vi "Test Dashboard.vi"() -> ()   [LabVIEW 2016]
uses:
  Program Files (x86)/National Instruments/LabVIEW 2016/examples/robotics/EPOS2 CANOpen Driver/Low Level VIs/Typedefs/FPGA CAN Frame Cluster.ctl
  BMS Status.ctl
  RT/Battery Status.ctl
  <vilib>/Utility/miscctls.llb/LVRowAndColumnUnsignedTypeDef.ctl
  <vilib>/Platform/TimedLoop/XDataNode/timing_clust.ctl
  <vilib>/Platform/TimedLoop/XDataNode/nitl_modes.ctl
  <vilib>/Platform/TimedLoop/XDataNode/wakeup.ctl
  RT/Read All CAN.vi
  RT/Data to BMS Status.vi
  RT/Data to Battery Status.vi
  <vilib>/Platform/TimedLoop/XDataNode/XDataNode.xnode
  <vilib>/Platform/TimedLoop/XDataNode/XDNodeRunTimeDep.lvlib
panel:
  in  "Tab Control":enum32{"Play!", "Debugg"}(tab)
  in  "Boot into load sequence":bool
  in  "No load":bool
  in  "Enter Stage":bool
  in  "Enter precharge":bool
  out "BMS Status":T1
  out "Stage req status":u8[](array[numeric])
  out "Stage req updates":u16
  out "Errors updates":u16
  out "Errors":u8[][](array[numeric]) format="%x"
  out "Battery Status":T2
  in  "CAN Frame":T3={"Timestamp"=0, "Identifier"=0, "Type"=0, "InfoA"=0, "InfoB"=0, "DataLength"=0, "Data"=[0, 0, 0, 0, 0, 0, 0, 0]} {"Data" format="%.0x"; "DataLength" format="%.0x"; "InfoB" format="%.0x"; "InfoA" format="%.0x"; "Type" format="%.0x"; "Identifier" format="%.0x"; "Timestamp" format="%.0x"}
  in  "Send once":bool
  in  "Send cont.":bool
  in  "Stop":bool
  out "Error Out":errorcluster
  out "CAN Frame Out":T3 {"Data" format="%.0x"; "DataLength" format="%.0x"; "InfoB" format="%.0x"; "InfoA" format="%.0x"; "Type" format="%.0x"; "Identifier" format="%.0x"; "Timestamp" format="%.0x"}
  in  "Clear list":bool
  out "Multicolumn Listbox":i32(listbox)
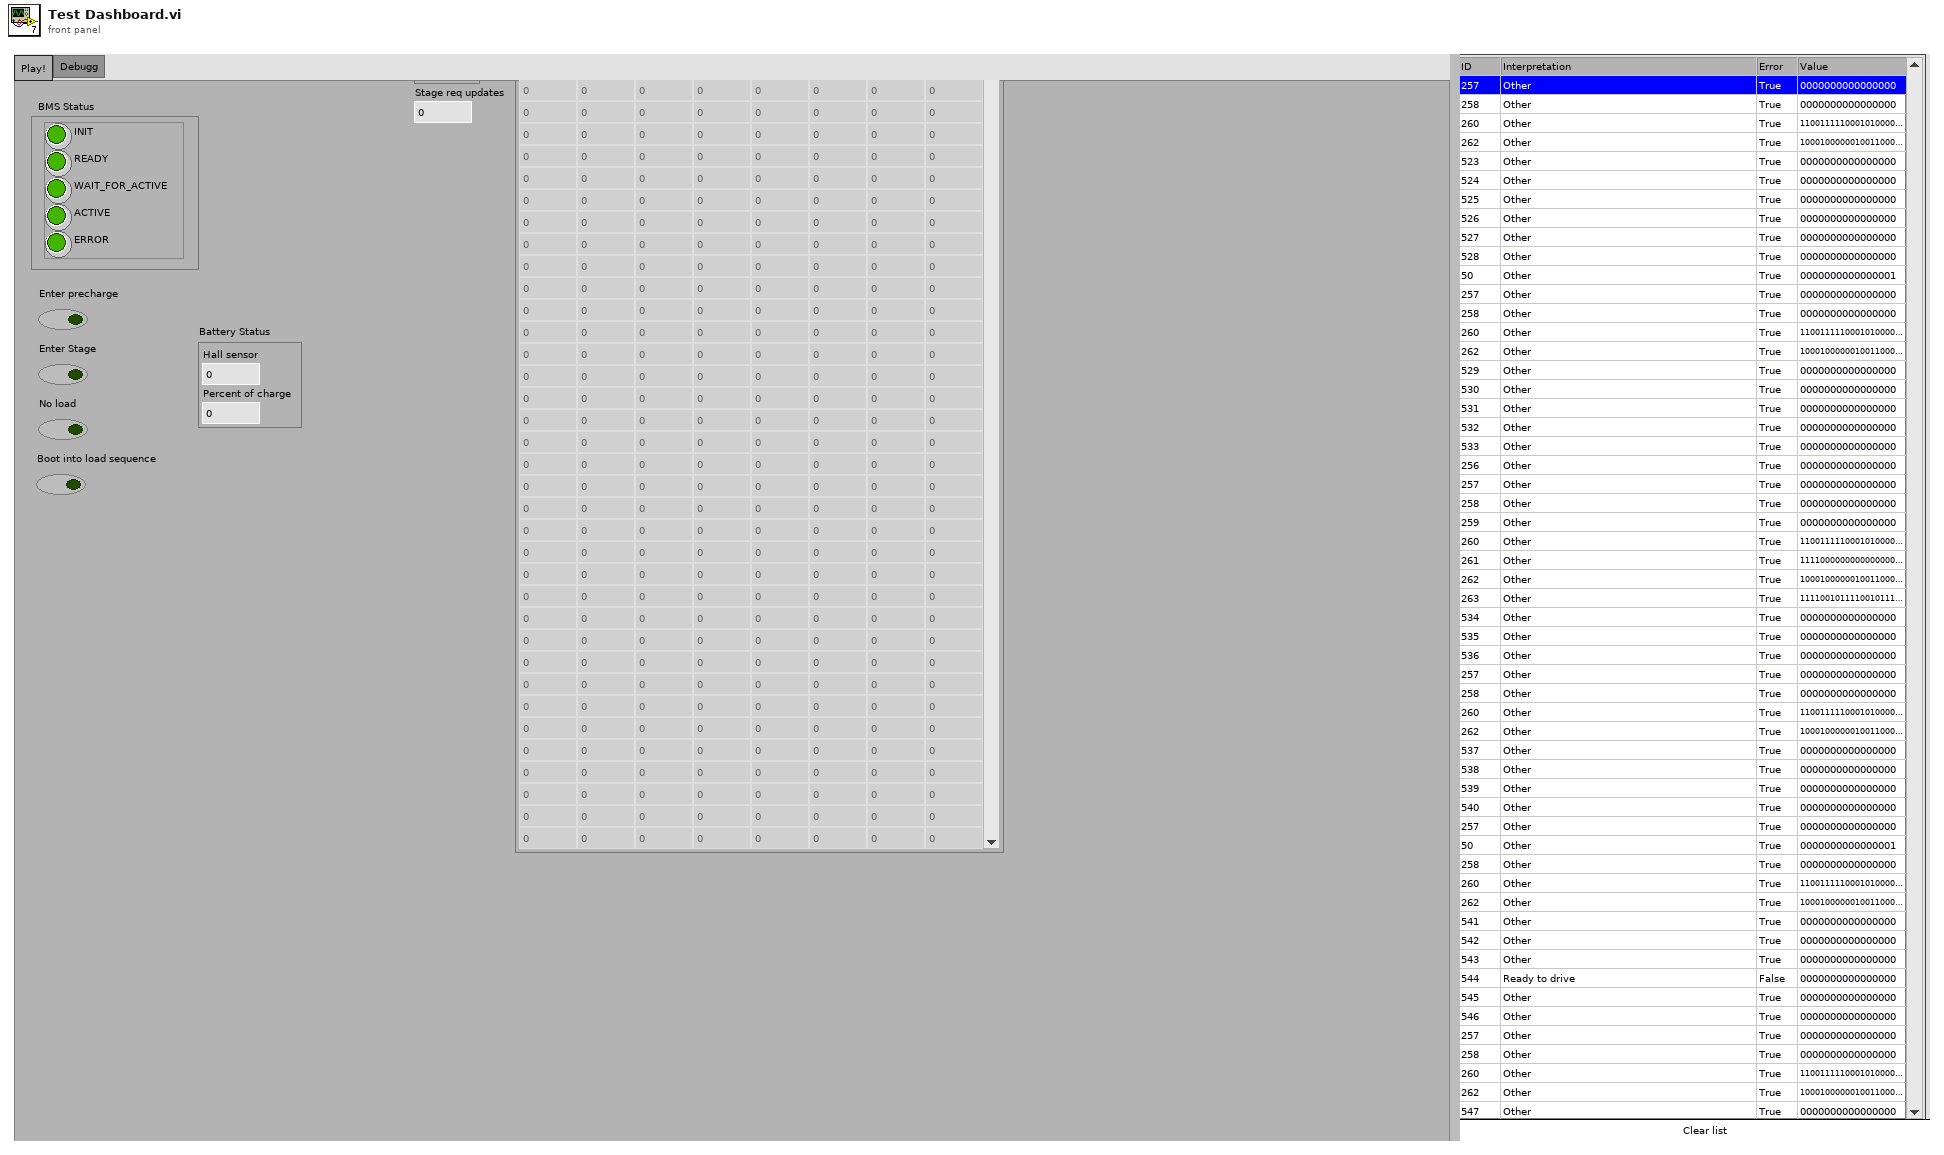
[diagram p1: front panel]
types:
  T1 = typedef "BMS Status.ctl" = cluster{"INIT":bool, "READY":bool, "WAIT_FOR_ACTIVE":bool, "ACTIVE":bool, "ERROR":bool}
  T2 = typedef "Battery Status.ctl" = cluster{"Hall sensor":i32, "Percent of charge":i16}
  T3 = typedef "FPGA CAN Frame Cluster.ctl" = cluster{"Timestamp":u64, "Identifier":u32, "Type":u8, "InfoA":u8, "InfoB":u8, "DataLength":u8, "Data":u8[]}
  T4 = cluster{"Message":string, "ID":u16, "Error":bool}[]
  T5 = typedef "XDNodeRunTimeDep.lvlib/timing_clust.ctl" = cluster{"Expected End [f-1]":u64, "Actual End [f-1]":u64, "Finished Late? [f-1]":bool, "Expected End [i-1]":u64, "Actual End [i-1]":u64, "Finished Late? [i-1]":bool, "Expected Start [i]":u64, "Actual Start [i]":u64, "Expected Start [f]":u64, "Actual Start [f]":u64, "Source Name":string, "Structure Name":string, "Period":i64, "Deadline":i64, "Offset":i64, "Start":i64, "Priority":i32, "Timeout":i32, "Mode":T6, "Wakeup Reason":T7, "Error":errorcluster, "Source Type":string, "Secondary Source Type":string, "Global End Time":u64, "Global Start Time":u64, "Frame Duration":u64, "Iteration Duration":u64, "Assigned CPU":i32, "I/O Scan Engine Mode":u32}
  T6 = typedef "XDNodeRunTimeDep.lvlib/nitl_modes.ctl" = enum32{"No Change", "Process missed periods, maintain original phase", "Discard missed periods, maintain original phase", "Process missed periods, ignore original phase", "Discard missed periods, ignore original phase"}
  T7 = typedef "XDNodeRunTimeDep.lvlib/wakeup.ctl" = enum32{"Normal", "Aborted", "Asynchronous wakeup", "Timing source error", "Timed loop error", "Timeout"}
  T8 = typedef "LVRowAndColumnUnsignedTypeDef.ctl" = cluster{"Row":u32, "Column":u32}
  T9 = typedef "CAN Refnum.ctl" = refnum<k1>
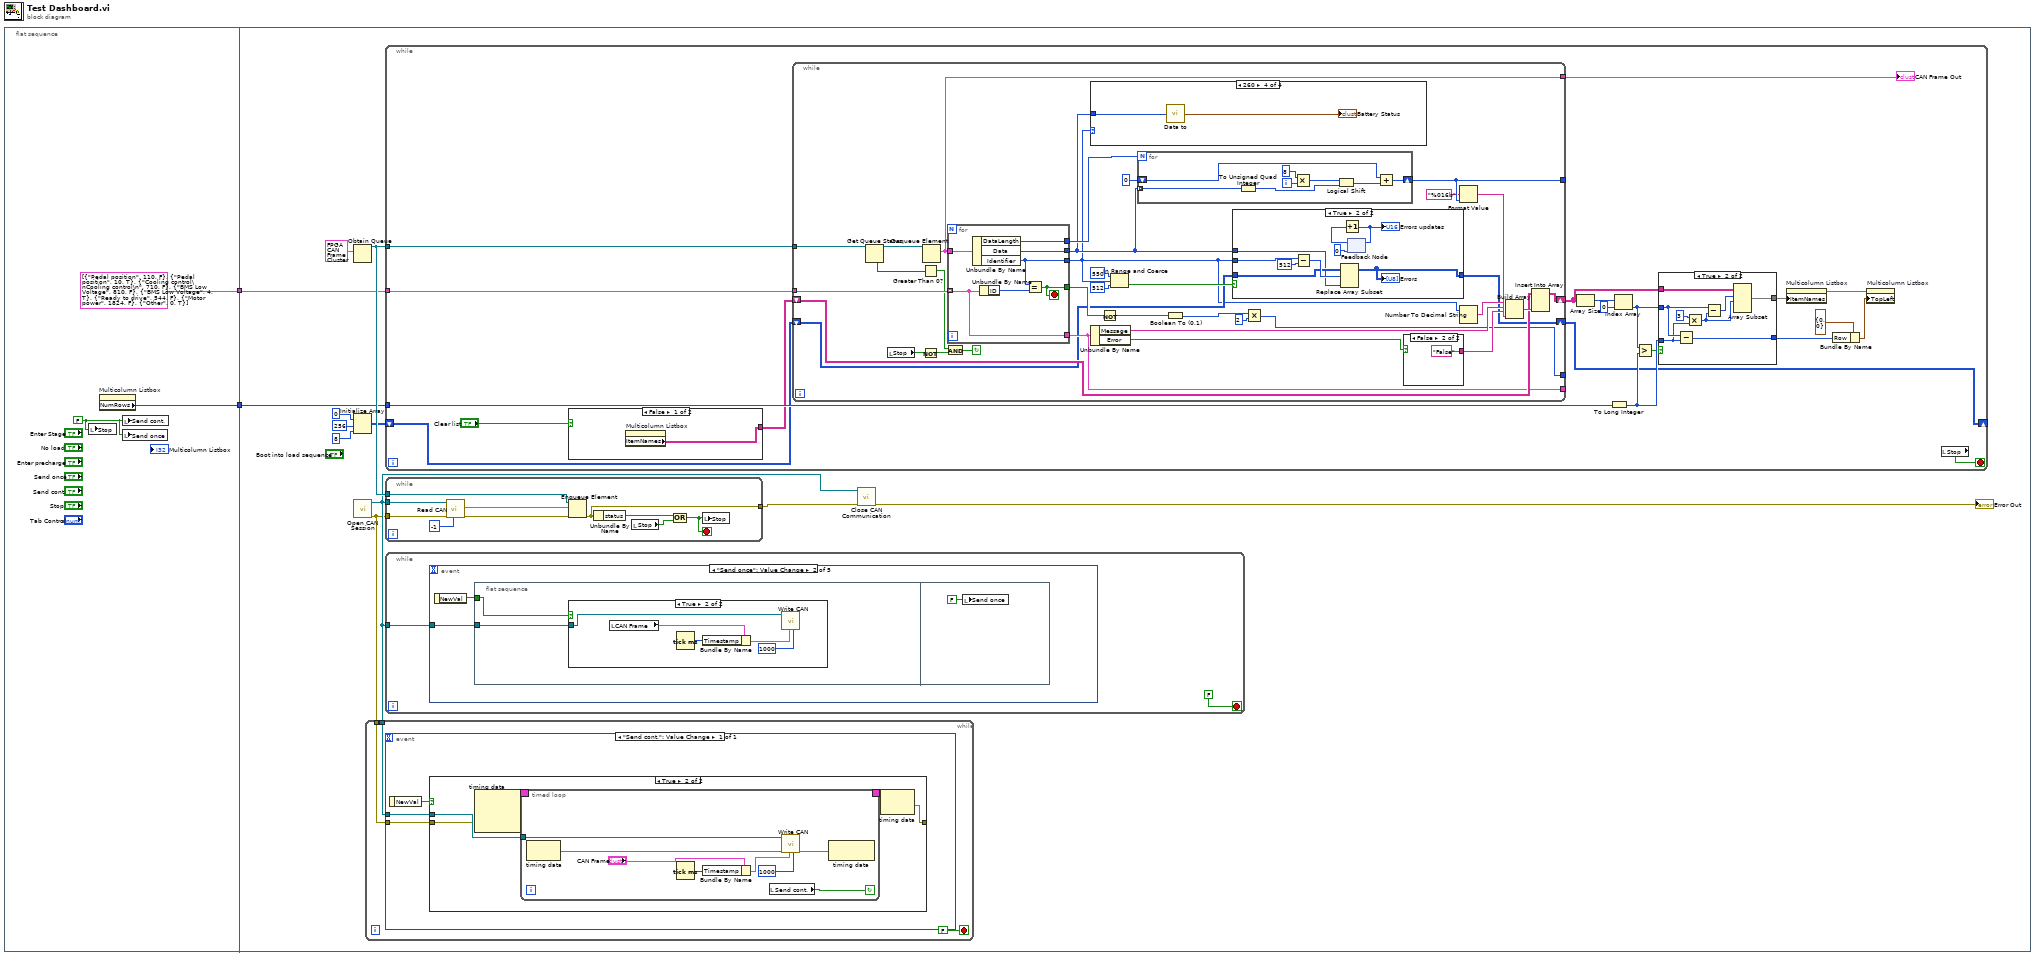
[diagram p0: block diagram]
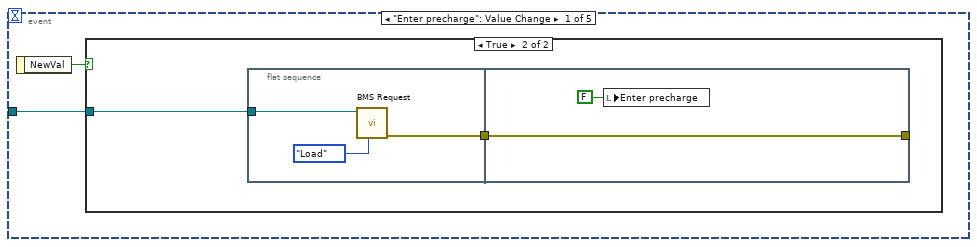
[diagram p3: hidden frame]
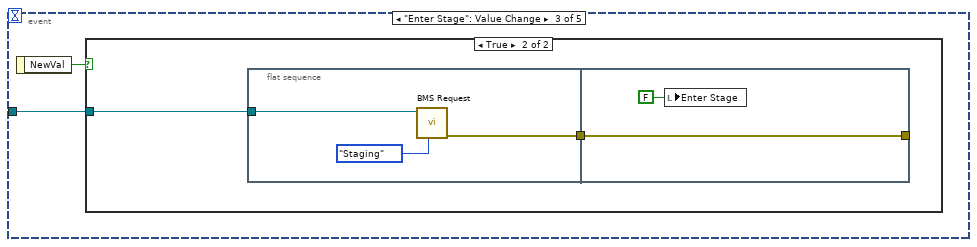
[diagram p6: hidden frame]
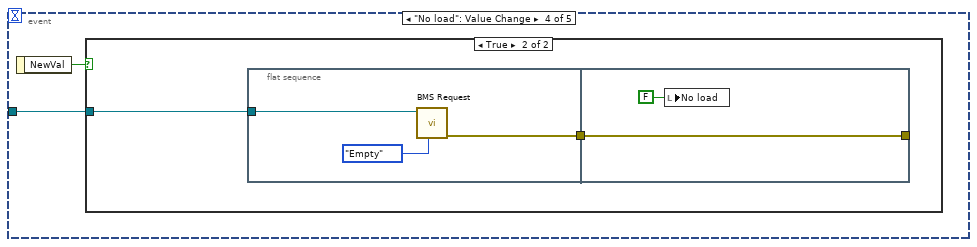
[diagram p8: hidden frame]
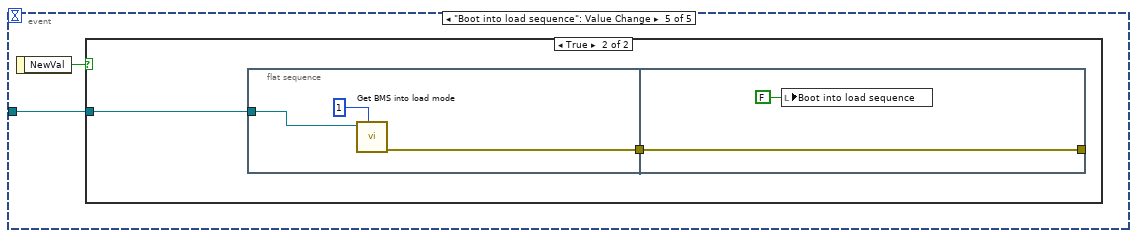
[diagram p10: hidden frame]
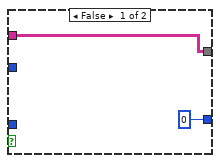
[diagram p12: hidden frame]
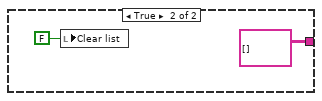
[diagram p13: hidden frame]
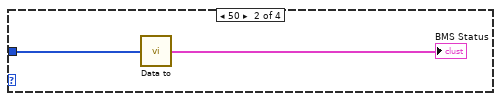
[diagram p16: hidden frame]
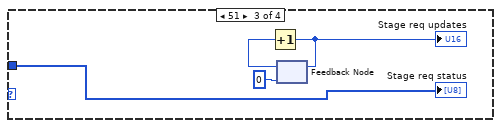
[diagram p17: hidden frame]
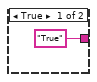
[diagram p18: hidden frame]
diagram:
  n1 = flat-sequence {
    tunnel: [w4] -> w2
    tunnel: [T4 [{"Message"="Pedal position", "ID"=110, "Error"=FALSE}, {"Message"="Pedal position", "ID"=10, "Error"=TRUE}, {"Message"="Cooling control\nCooling control\n", "ID"=710, "Error"=FALSE}, {"Message"="BMS Low Voltage", "ID"=810, "Error"=FALSE}, {"Message"="BMS Low Voltage", "ID"=4, "Error"=TRUE}, {"Message"="Ready to drive", "ID"=544, "Error"=FALSE}, {"Message"="Motor power", "ID"=1824, "Error"=FALSE}, {"Message"="Other", "ID"=0, "Error"=TRUE}] ("Messages")] -> w1
    tunnel: w2 -> [w14]
    tunnel: w1 -> [w13]
    frame #0 {
      w5 = FALSE
      n2 = local write "Stop"(w5) -> ()
      n3 = property on="Multicolumn Listbox" class="MCListbox (strict)"() -> ("NumRows"=w4:u32)  [unwired: 2 in, 2 out]
      n4 = local write "Send cont."(w5) -> ()
      n5 = local write "Send once"(w5) -> ()
    }
    frame #1 {
      n6 = Initialize Array(u8 0 ("element"), 256 ("dimension size"), 8 ("dimension size")) -> (w9:u8[][])
      n7 = Obtain Queue(element data type=T3 {"Timestamp"=0, "Identifier"=0, "Type"=0, "InfoA"=0, "InfoB"=0, "DataLength"=0, "Data"=[0, 0, 0, 0, 0, 0, 0, 0]} ("CAN Frame Out")) -> (queue out=w16:refnum<queue>)  [unwired: 4 in, 2 out]
      n8 = call "Open CAN Session.vi"() -> ("error out"=w6:errorcluster, "CAN Session"=w7:T9)  [unwired: 10 in]
      n9 = while {
        tunnel: w7 -> [w20]
        tunnel: w6 -> [w19]
        stop <- FALSE stop-if-true
        n10 = event shown="[0] \"Send cont.\": Value Change" {
          selector: _ -> [_]
          dyn-events: _ -> [_]
          timeout: _ -> [_]
          tunnel: w20 -> [w22]
          tunnel: w19 -> [w21]
          event "Send cont.": Value Change {
            n11 = event-data() -> ("NewVal"=w23:bool)  [unwired: 1 in]
            n12 = case shown="True" w23 {
              tunnel: w21 -> [w24 w26]
              tunnel: w22 -> [_ w27]
              tunnel: [w24 w25] -> _
              frame False {
              }
              frame True {
                n13 = node-c288(w26) -> (w29:T5)  [unwired: 2 in]
                n14 = timed-loop {
                  timing: w29 -> [_]
                  timing-out: [_] -> w28
                  tunnel: w27 -> [w37]
                  stop <- w34 continue-if-true
                  n15 = node-c288() -> (w36:errorcluster)  [unwired: 1 in]
                  n16 = Tick Count (ms)() -> (millisecond timer value=w30:u32)
                  n17 = Bundle By Name(cluster="CAN Frame", "Timestamp"=w30) -> (w31:T3)
                  n18 = local read "Send cont."() -> (w34:bool)
                  n19 = call "Write CAN.vi"("timeout"=1000, "CAN Frame"=w31, "error in"=w36, "CAN Session In"=w37) -> ("error out"=w35:errorcluster)  [unwired: 6 in, 1 out]
                  n20 = node-c288(w35) -> ()  [unwired: 1 out]
                }
                n21 = node-c288(w28) -> (w25:errorcluster)
              }
            }
          }
        }
      }
      n22 = while {
        tunnel: w16 -> [w115]
        tunnel: w14 -> [w109]
        tunnel: w13 -> [w108]
        shift-right: [w96] -> _
        shift-left: w9 -> [w97]
        stop <- w113 stop-if-true
        n23 = case shown="False" "Clear list" {
          tunnel: [w126 string[][] [] ("Item Names")] -> w106
          frame False {
            n24 = property on="Multicolumn Listbox" class="MCListbox (strict)"() -> ("ItemNames"=w126:string[][])  [unwired: 2 in, 2 out]
          }
          frame True {
            n25 = local write "Clear list"(FALSE) -> ()
          }
        }
        n26 = while {
          tunnel: w115 -> [w160]
          tunnel: [w145] -> _
          tunnel: [w137] -> _
          tunnel: [w144] -> w114
          tunnel: [w143] -> _
          shift-right: [w146] -> w102
          shift-left: w106 -> [w147]
          tunnel: w108 -> [w142]
          shift-right: [w131] -> w96
          shift-left: w97 -> [w132]
          stop <- w138 continue-if-true
          n27 = Get Queue Status(queue=w160) -> (queue out=w161:refnum<queue>, # elements in queue=w162:i32)  [unwired: 2 in, 6 out]
          n28 = local read "Stop"() -> (w141:bool)
          n29 = Greater Than 0?(x=w162) -> (x > 0?=w139:bool)
          n30 = Not(x=w141) -> (.not. x?=w140:bool)
          n31 = Dequeue Element(queue=w161) -> (element=w144:T3)  [unwired: 2 in, 3 out]
          n32 = And(x=w139, y=w140) -> (x .and. y?=w138:bool)
          n33 = for {
            tunnel: w142 -> [w195] mode=indexing
            tunnel: w144 -> [w197]
            tunnel: [w195] -> w143
            tunnel: [w194] -> w149
            tunnel: [w193] -> w130
            tunnel: [w192] -> w148
            tunnel: [w191] -> w129
            stop <- w194 stop-if-true
            n34 = Unbundle By Name(w197) -> ("DataLength"=w192:u8, "Data"=w193:u8[], "Identifier"=w191:u32)
            n35 = Unbundle By Name(w195) -> ("ID"=w196:u16)
            n36 = Equal?(x=w191, y=w196) -> (x = y?=w194:bool)
          }
          n37 = case shown="260" w129 {
            tunnel: w130 -> [_ w174 w178 w180]
            frame 0, Default {
            }
            frame 50 {
              n38 = call-poly "Data to.vi"("Data"=w174) -> ("BMS Status"=→"BMS Status":T1)
            }
            frame 51 {
              n39 = feedback #1(u16 0) -> (w177:u16)
              n40 = Increment(x=w177) -> (x+1=w176:u16)
              "Stage req updates" <- w176
              n41 = feedback-in #1(w176) -> ()
              "Stage req status" <- w178
            }
            frame 260 {
              n42 = call-poly "Data to.vi"("Data"=w180) -> ("Battery Status"=→"Battery Status":T2)
            }
          }
          n43 = Unbundle By Name(w143) -> ("Message"=w153:string, "Error"=w155:bool)
          n44 = Not(x=w149) -> (.not. x?=w152:bool)
          n45 = In Range and Coerce(upper limit=u16 550, x=w129, lower limit=u16 512) -> (In Range?=w133:bool)  [unwired: 1 out]
          n46 = for {
            N: w148 -> [_]
            shift-right: [w182] -> w137
            shift-left: u64 0 -> [w184]
            tunnel: w130 -> [w181] mode=indexing
            i -> [w186]
            n47 = To Unsigned Quad Integer(1:w181) -> (0:w183:u64)
            n48 = Multiply(x=i8 8, y=w186) -> (x*y=w185:i32)
            n49 = Logical Shift(y=w185, x=w183) -> (x << y=w188:u64)
            n50 = Add(x=w184, y=w188) -> (x+y=w182:u64)
          }
          n51 = Boolean To (0,1)(Boolean=w152) -> (0, 1=w150:i16)
          n52 = case shown="True" w133 {
            tunnel: w132 -> [w163 w167]
            tunnel: [w163 w166] -> w131
            tunnel: w130 -> [_ w165]
            tunnel: w129 -> [_ w164]
            frame False {
            }
            frame True {
              n53 = Subtract(x=w164, y=u32 512) -> (x-y=w172:u32)
              n54 = Replace Array Subset(array=w167, new element=w165, index (row)=w172) -> (w166:u8[][])  [unwired: 1 in]
              "Errors" <- w166
              n55 = feedback #2(u16 0) -> (w168:u16)
              n56 = Increment(x=w168) -> (x+1=w169:u16)
              "Errors updates" <- w169
              n57 = feedback-in #2(w169) -> ()
            }
          }
          n58 = Multiply(x=w150, y=i16 2) -> (x*y=w145:i16)
          n59 = case shown="False" w155 {
            tunnel: ["True" "False"] -> w156
            frame True {
            }
            frame False {
            }
          }
          n60 = Format Value(format string="%016b", value (0)=w137) -> (output string=w158:string)  [unwired: 1 in]
          n61 = Number To Decimal String(number=w129) -> (decimal integer string=w154:string)  [unwired: 1 in]
          n62 = Build Array(w154, w153, w156, w158) -> (w157:string[])
          n63 = Insert Into Array(array=w147, new element=w157) -> (w146:string[][])  [unwired: 2 in]
        }
        "CAN Frame Out" <- w114
        n64 = Array Size(array=w102) -> (size(s)=w104:i32[])
        n65 = To Long Integer(number=w109) -> (32bit integer=w99:i32)
        n66 = Index Array(array=w104, index=0) -> (element=w100:i32)
        n67 = Greater?(x=w100, y=w99) -> (0:w98:bool)
        n68 = case shown="True" w98 {
          tunnel: [0 w118] -> w103
          tunnel: w99 -> [_ w119]
          tunnel: w100 -> [_ w120]
          tunnel: w102 -> [w116 w123]
          tunnel: [w116 w122] -> w101
          frame False {
          }
          frame True {
            n69 = Subtract(x=w120, y=w119) -> (x-y=w118:i32)
            n70 = Multiply(x=3, y=w119) -> (x*y=w124:i32)
            n71 = Subtract(x=w120, y=w124) -> (x-y=w125:i32)
            n72 = Array Subset(array=w123, index (row)=w125, length (row)=w124) -> (w122:string[][])  [unwired: 2 in]
          }
        }
        n73 = property on="Multicolumn Listbox" class="MCListbox (strict)"("ItemNames"=w101) -> (error out=w105:errorcluster)  [unwired: 2 in, 1 out]
        n74 = Bundle By Name(cluster=T8 {"Row"=0, "Column"=0} ("Top Left Visible Cell"), "Row"=w103) -> (w112:T8)
        n75 = property on="Multicolumn Listbox" class="MCListbox (strict)"(error in=w105, "TopLeft"=w112) -> ()  [unwired: 1 in, 2 out]
        n76 = local read "Stop"() -> (w113:bool)
      }
      n77 = while {
        tunnel: w6 -> [w199]
        tunnel: w7 -> [w198]
        tunnel: w16 -> [w205]
        tunnel: [w203] -> w15
        stop <- w206 stop-if-true
        n78 = call-poly "Read CAN.vi"("timeout in ms (-1)"=-1, "error in"=w199, "CAN Session In"=w198) -> ("error out"=w201:errorcluster, "CAN Frame Out"=w202:T3)  [unwired: 6 in, 1 out]
        n79 = Enqueue Element(queue=w205, element=w202, error in (no error)=w201) -> (error out=w203:errorcluster)  [unwired: 1 in, 2 out]
        n80 = Unbundle By Name(w203) -> ("status"=w204:bool)
        n81 = local read "Stop"() -> (w207:bool)
        n82 = Or(x=w204, y=w207) -> (x .or. y?=w206:bool)
        n83 = local write "Stop"(w206) -> ()
      }
      n84 = while {
        tunnel: w7 -> [w49]
        stop <- FALSE stop-if-true
        n85 = event shown="[1] \"Send once\": Value Change" {
          selector: _ -> [_ _ _ _ _]
          dyn-events: _ -> [_ _ _ _ _]
          timeout: _ -> [_ _ _ _ _]
          tunnel: w49 -> [w51 w59 w70 w79 w88]
          event "Enter precharge": Value Change {
            n86 = event-data() -> ("NewVal"=w50:bool)  [unwired: 1 in]
            n87 = case shown="True" w50 {
              tunnel: w51 -> [_ w52]
              frame False {
              }
              frame True {
                n88 = flat-sequence {
                  tunnel: [w55] -> w53
                  tunnel: w52 -> [w56]
                  tunnel: [w58] -> _
                  tunnel: w53 -> [w58]
                  frame #0 {
                    n89 = call "BMS Request.vi"("Request"=enum16{"Empty", "Load", "Staging"}."Load", "CAN Session In"=w56) -> ("error out"=w55:errorcluster)  [unwired: 8 in, 1 out]
                  }
                  frame #1 {
                    n90 = local write "Enter precharge"(FALSE) -> ()
                  }
                }
              }
            }
          }
          event "Send once": Value Change {
            n91 = event-data() -> ("NewVal"=w60:bool)  [unwired: 1 in]
            n92 = flat-sequence {
              tunnel: w60 -> [w62]
              tunnel: w59 -> [w61]
              frame #0 {
                n93 = case shown="True" w62 {
                  tunnel: w61 -> [_ w63]
                  frame False {
                  }
                  frame True {
                    n94 = local read "CAN Frame"() -> (w64:T3)
                    n95 = Tick Count (ms)() -> (millisecond timer value=w65:u32)
                    n96 = Bundle By Name(cluster=w64, "Timestamp"=w65) -> (w66:T3)
                    n97 = call "Write CAN.vi"("timeout"=1000, "CAN Frame"=w66, "CAN Session In"=w63) -> ()  [unwired: 7 in, 2 out]
                  }
                }
              }
              frame #1 {
                n98 = local write "Send once"(FALSE ("Send once")) -> ()
              }
            }
          }
          event "Enter Stage": Value Change {
            n99 = event-data() -> ("NewVal"=w69:bool)  [unwired: 1 in]
            n100 = case shown="True" w69 {
              tunnel: w70 -> [_ w71]
              frame False {
              }
              frame True {
                n101 = flat-sequence {
                  tunnel: [w74] -> w72
                  tunnel: w71 -> [w75]
                  tunnel: [w77] -> _
                  tunnel: w72 -> [w77]
                  frame #0 {
                    n102 = call "BMS Request.vi"("Request"=enum16{"Empty", "Load", "Staging"}."Staging", "CAN Session In"=w75) -> ("error out"=w74:errorcluster)  [unwired: 8 in, 1 out]
                  }
                  frame #1 {
                    n103 = local write "Enter Stage"(FALSE) -> ()
                  }
                }
              }
            }
          }
          event "No load": Value Change {
            n104 = event-data() -> ("NewVal"=w78:bool)  [unwired: 1 in]
            n105 = case shown="True" w78 {
              tunnel: w79 -> [_ w80]
              frame False {
              }
              frame True {
                n106 = flat-sequence {
                  tunnel: [w83] -> w81
                  tunnel: w80 -> [w84]
                  tunnel: [w86] -> _
                  tunnel: w81 -> [w86]
                  frame #0 {
                    n107 = call "BMS Request.vi"("Request"=enum16{"Empty", "Load", "Staging"}."Empty", "CAN Session In"=w84) -> ("error out"=w83:errorcluster)  [unwired: 8 in, 1 out]
                  }
                  frame #1 {
                    n108 = local write "No load"(FALSE) -> ()
                  }
                }
              }
            }
          }
          event "Boot into load sequence": Value Change {
            n109 = event-data() -> ("NewVal"=w87:bool)  [unwired: 1 in]
            n110 = case shown="True" w87 {
              tunnel: w88 -> [_ w89]
              frame False {
              }
              frame True {
                n111 = flat-sequence {
                  tunnel: [w91] -> w90
                  tunnel: w89 -> [w93]
                  tunnel: [w95] -> _
                  tunnel: w90 -> [w95]
                  frame #0 {
                    n112 = call "Get BMS into load mode.vi"("timeout in ms (-1)"=1, "CAN Session In"=w93) -> ("error out"=w91:errorcluster)  [unwired: 7 in, 2 out]
                  }
                  frame #1 {
                    n113 = local write "Boot into load sequence"(FALSE) -> ()
                  }
                }
              }
            }
          }
        }
      }
      n114 = call "Close CAN Communication.vi"("error in"=w15, "CAN Session"=w7) -> ("error out"=→"Error Out":errorcluster)  [unwired: 9 in]
    }
  }
